vi "Quadratic Formula Fixed.vi"() -> ()   [LabVIEW 2015]
doc: "This VI plots and solves a quadratic equation."
panel:
  out "XY Graph":cluster{dbl, dbl}[](graph)
  out "Answer 2":dbl
  out "Answer 1":dbl
  in  "C":dbl
  in  "B":dbl
  in  "A":dbl
  # "Y = a*X^2 + b*X + c"
  # "Finds the values of X when Y = 0"
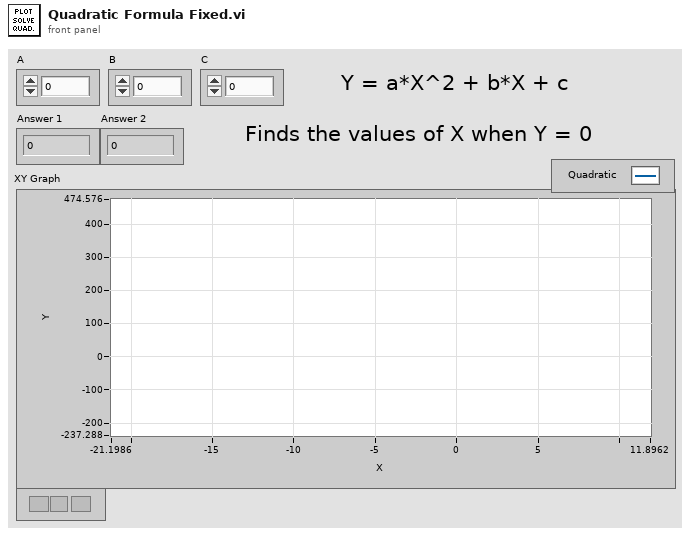
[diagram p1: front panel]
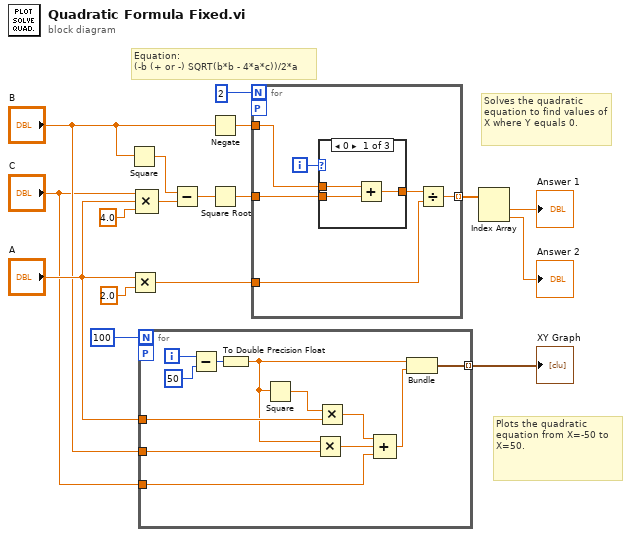
[diagram p0: block diagram]
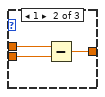
[diagram p2: hidden frame]
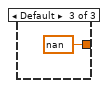
[diagram p3: hidden frame]
diagram:
  # "Equation:\n(-b (+ or -) SQRT(b*b - 4*a*c))/2*a"
  # "Plots the quadratic equation from X=-50 to X=50."
  # "Solves the quadratic equation to find values of X where Y equals 0."
  n1 = Square(x="B") -> (x^2=w4:dbl)
  n2 = Multiply(x="A", y=2.0) -> (x*y=w10:dbl)
  n3 = Compound Arithmetic op=MULTIPLY("C", "A", 4.0 ("value")) -> (w14:dbl)
  n4 = for {
    N: 100 -> [_]
    tunnel: "A" -> [w26]
    tunnel: "B" -> [w25]
    tunnel: "C" -> [w22]
    tunnel: [w19] -> w5 mode=indexing
    workers-P: _ -> [_]
    i -> [w29]
    n5 = Subtract(x=w29, y=50) -> (x-y=w21:i32)
    n6 = To Double Precision Float(number=w21) -> (double precision float=w18:dbl)
    n7 = Square(x=w18) -> (x^2=w27:dbl)
    n8 = Multiply(x=w18, y=w25) -> (x*y=w23:dbl)
    n9 = Multiply(x=w27, y=w26) -> (x*y=w24:dbl)
    n10 = Compound Arithmetic op=ADD(w24, w23, w22) -> (w20:dbl)
    n11 = Bundle(w18, w20) -> (w19:cluster{dbl, dbl})  [unwired: 1 in]
  }
  "XY Graph" <- w5
  n12 = Subtract(x=w4, y=w14) -> (x-y=w13:dbl)
  n13 = Negate(x="B") -> (-x=w12:dbl)
  n14 = Square Root(x=w13) -> (sqrt(x)=w9:dbl)
  n15 = for {
    N: 2 -> [_]
    tunnel: w12 -> [w35]
    tunnel: w10 -> [w34]
    tunnel: w9 -> [w33]
    tunnel: [w30] -> w7 mode=indexing
    workers-P: _ -> [_]
    i -> [w31]
    n16 = case shown="0" w31 {
      tunnel: w35 -> [w38 w41 _]
      tunnel: w33 -> [w37 w40 _]
      tunnel: [w36 w39 nan] -> w32
      frame 0 {
        n17 = Add(x=w38, y=w37) -> (x+y=w36:dbl)
      }
      frame 1 {
        n18 = Subtract(x=w41, y=w40) -> (x-y=w39:dbl)
      }
      frame Default {
      }
    }
    n19 = Divide(x=w32, y=w34) -> (x/y=w30:dbl)
  }
  n20 = Index Array(array=w7) -> (element #1=→"Answer 1":dbl, element #2=→"Answer 2":dbl)  [unwired: 2 in]
